vi "OP500ZP_Softs.vi"(8 "errin":errorcluster caption="entrée d'erreur (pas d'erreur)") -> (0 "errout":errorcluster caption="error out", 3 "OUI/NON":bool)   [LabVIEW 2020]
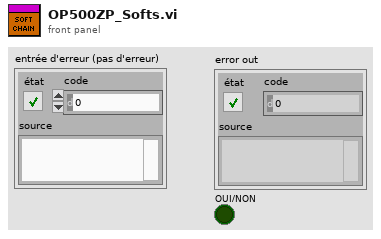
[diagram p1: front panel]
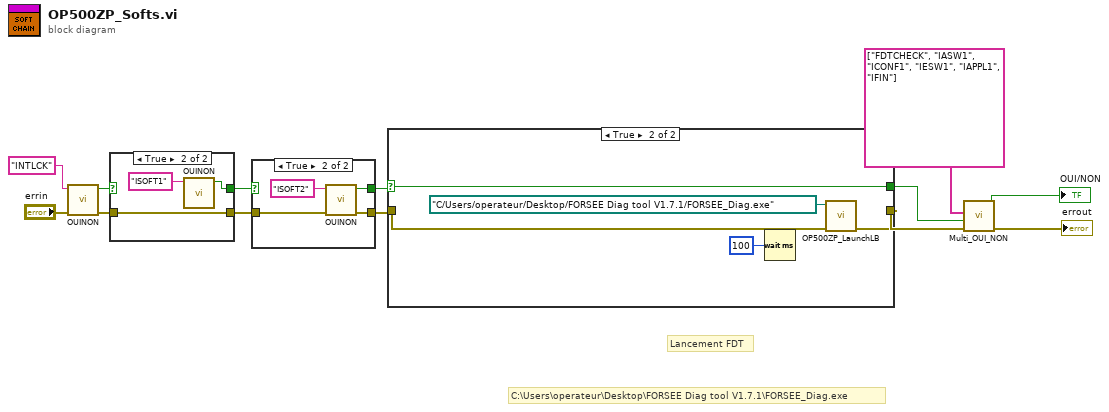
[diagram p0: block diagram]
diagram:
  # "C:\\Users\\operateur\\Desktop\\FORSEE Diag tool V1.7.1\\FORSEE_Diag.exe"
  # "Lancement FDT"
  n1 = call "OUINON.vi"("errin"="errin", "image"="INTLCK") -> ("error out"=w7:errorcluster, "OUI/NON"=w6:bool)  [unwired: 8 in]
  n2 = case shown="True" w6 {
    selector: w6 -> [w15 _]
    tunnel: [w15 w16] -> w10
    tunnel: [w14 w17] -> w11
    tunnel: w7 -> [w14 w17]
    frame False {
    }
    frame True {
      n3 = call "OUINON.vi"("image"="ISOFT1") -> ("OUI/NON"=w16:bool)  [unwired: 9 in, 1 out]
    }
  }
  n4 = case shown="True" w10 {
    selector: w10 -> [w19 _]
    tunnel: w11 -> [w20 w24]
    tunnel: [w19 w23] -> w13
    tunnel: [w20 w22] -> w12
    frame False {
    }
    frame True {
      n5 = call "OUINON.vi"("errin"=w24, "image"="ISOFT2") -> ("error out"=w22:errorcluster, "OUI/NON"=w23:bool)  [unwired: 8 in]
    }
  }
  n6 = case shown="True" w13 {
    selector: w13 -> [w25 w29]
    tunnel: w12 -> [w26 w31]
    tunnel: [w26 w30] -> w2
    tunnel: [w25 w29] -> w1
    frame False {
    }
    frame True {
      n7 = Wait (ms)(milliseconds to wait=u32 100 ("attente (ms)")) -> ()  [unwired: 1 out]
      n8 = call "OP500ZP_LaunchLB.vi"("errin"=w31, "Application à lancer"=path "C:/Users/operateur/Desktop/FORSEE Diag tool V1.7.1/FORSEE_Diag.exe") -> ("error out"=w30:errorcluster)  [unwired: 7 in]
    }
  }
  n9 = call "Multi_OUI_NON.vi"("errin"=w2, "errinb"=w1, "Tableau"=string[] ["FDTCHECK", "IASW1", "ICONF1", "IESW1", "IAPPL1", "IFIN"]) -> ("errout"=→"errout":errorcluster, "isok?"=→"OUI/NON":bool)  [unwired: 7 in]
